vi "Example.vi"() -> ()   [LabVIEW 2015]
uses:
  Signals.ctl
  <vilib>/LV-Signals/create-xnode/LV-Create-Signals.xnode
  <vilib>/LV-Signals/read-write-xnode/LV-Read-Write-Signals.xnode
  <vilib>/LV-Signals/destroy-xnode/LV-Destroy-Signals.xnode
panel:
  out "String":string
  in  "Number":dbl=5.0 format="%#_13g"
  out "Values":T1
  in  "String":string
  in  "Array Index 2":i32=1
  in  "Array Index":i32
  in  "Stop Button":bool
  out "Array":cluster{"Array":cluster{"Number":dbl}[]}[](array[cluster])
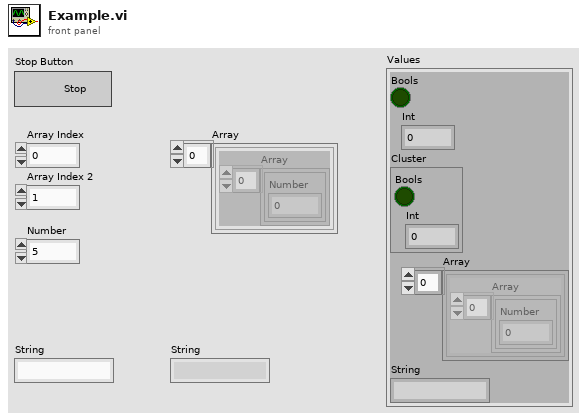
[diagram p1: front panel]
types:
  T1 = cluster{"Bools":bool, "Int":i32, "Cluster":cluster{"Bools":bool, "Int":i32}, "Array":cluster{"Array":cluster{"Number":dbl}[]}[], "String":string}
  T2 = typedef "Signals.ctl" = cluster{"DVR":refnum<data-value>, "Module Events":cluster{"Bools":refnum<user-event>, "Int":refnum<user-event>, "Cluster":refnum<user-event>, "Array":refnum<user-event>, "String":refnum<user-event>}}
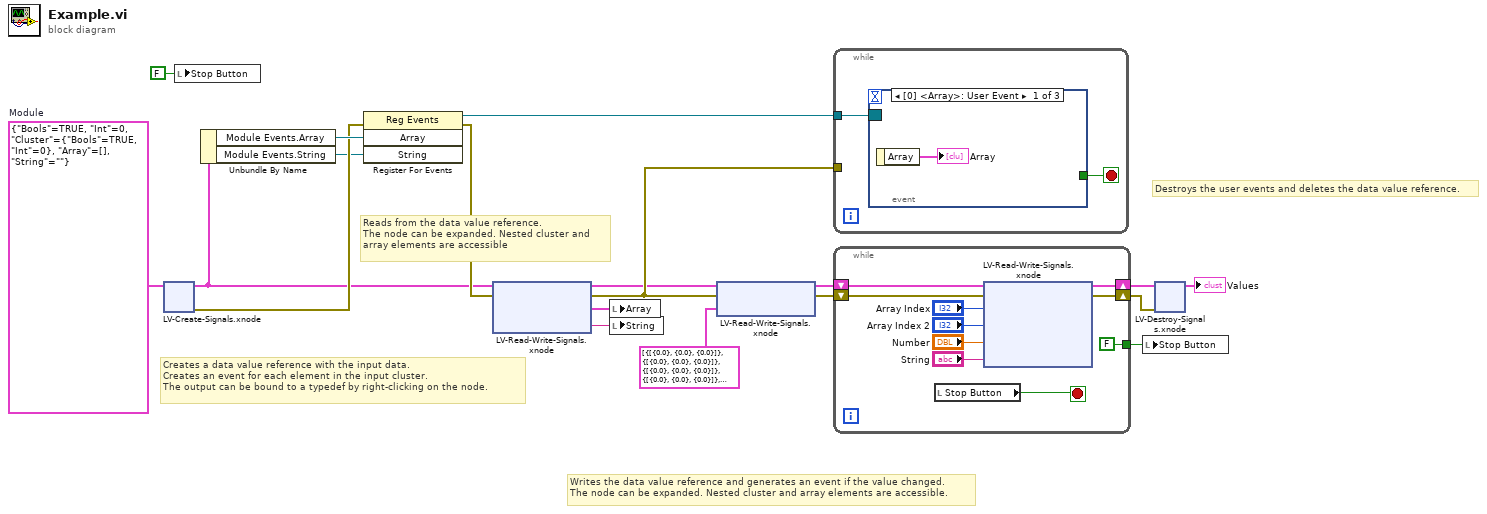
[diagram p0: block diagram]
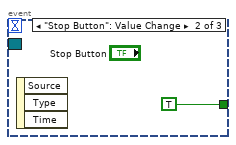
[diagram p2: hidden frame]
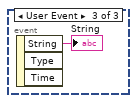
[diagram p3: hidden frame]
diagram:
  w13 = T1 {"Bools"=TRUE, "Int"=0, "Cluster"={"Bools"=TRUE, "Int"=0}, "Array"=[], "String"=""}  # Module
  # "Destroys the user events and deletes the data value reference."
  # "Writes the data value reference and generates an event if the value changed.\nThe node can be expanded. Nested cluster and array elements are accessible."
  # "Reads from the data value reference.\nThe node can be expanded. Nested cluster and\narray elements are accessible"
  # "Creates a data value reference with the input data.\nCreates an event for each element in the input cluster.\nThe output can be bound to a typedef by right-clicking on the node."
  n1 = xnode "LV-Create-Signals.xnode"("Values"=w13) -> ("Signals"=w4:T2, "Error Out"=w16:errorcluster)  [unwired: 1 in]
  n2 = local write "Stop Button"(FALSE ("Stop Button")) -> ()
  n3 = Unbundle By Name(w4) -> ("Module Events.Array"=w17:refnum<user-event>, "Module Events.String"=w6:refnum<user-event>)
  n4 = register-events(error in=w16, w17, w6) -> (reference out=w14:refnum<event-registration>, error out=w15:errorcluster)  [unwired: 1 in]
  n5 = xnode "LV-Read-Write-Signals.xnode"("Signals In"=w4, "Error In"=w15) -> ("Signals Out"=w8:T2, "Error Out"=w11:errorcluster, "Array"=w3:cluster{"Array":cluster{"Number":dbl}[]}[], "String"=w2:string)
  n6 = local write "Array"(w3) -> ()
  n7 = local write "String"(w2) -> ()
  n8 = xnode "LV-Read-Write-Signals.xnode"("Signals In"=w8, "Error In"=w11, "Array"=cluster{"Array":cluster{"Number":dbl}[]}[] [{"Array"=[{"Number"=0.0}, {"Number"=0.0}, {"Number"=0.0}]}, {"Array"=[{"Number"=0.0}, {"Number"=0.0}, {"Number"=0.0}]}, {"Array"=[{"Number"=0.0}, {"Number"=0.0}, {"Number"=0.0}]}, {"Array"=[{"Number"=0.0}, {"Number"=0.0}, {"Number"=0.0}]}, {"Array"=[{"Number"=0.0}, {"Number"=0.0}, {"Number"=0.0}]}]) -> ("Signals Out"=w12:T2, "Error Out"=w10:errorcluster)
  n9 = while {
    tunnel: w14 -> [w21]
    tunnel: w11 -> [_]
    stop <- w20 stop-if-true
    n10 = event shown="[0] <Array>: User Event" {
      selector: w21 -> [_ _ _]
      dyn-events: _ -> [_ _ _]
      timeout: _ -> [_ _ _]
      tunnel: [_ TRUE _] -> w20
      event User Event {
        n11 = event-data() -> ("Array"=→"Array":cluster{"Array":cluster{"Number":dbl}[]}[])  [unwired: 1 in]
      }
      event "Stop Button": Value Change {
        n12 = event-data() -> ()  [unwired: 1 in, 3 out]
      }
      event User Event {
        n13 = event-data() -> ("String"=→"String":string)  [unwired: 1 in, 2 out]
      }
    }
  }
  n14 = while {
    shift-right: [w34] -> w19
    shift-left: w12 -> [w32]
    shift-right: [w33] -> w18
    shift-left: w10 -> [w31]
    tunnel: [FALSE] -> w7
    stop <- w30 stop-if-true
    n15 = local read "Stop Button"() -> (w30:bool)
    n16 = xnode "LV-Read-Write-Signals.xnode"("Signals In"=w32, "Error In"=w31, "Array[]"="Array Index", "Element.Array[]"="Array Index 2", "Element.Number"="Number", "String"="String") -> ("Signals Out"=w34:T2, "Error Out"=w33:errorcluster)
  }
  n17 = local write "Stop Button"(w7) -> ()
  n18 = xnode "LV-Destroy-Signals.xnode"("Signals"=w19, "Error In"=w18) -> ("Values"=→"Values":T1)  [unwired: 1 out]
